vi "General.vi"() -> ()   [LabVIEW 2023]
panel:
  in  "Stop Button":bool
  out "Boolean":bool
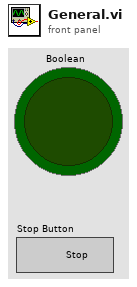
[diagram p1: front panel]
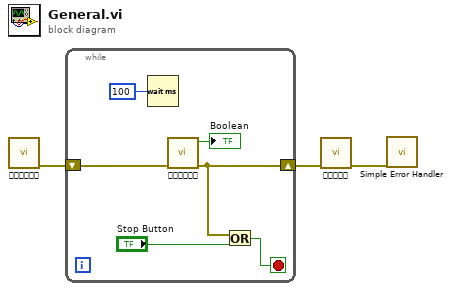
[diagram p0: block diagram]
diagram:
  n1 = call "설정.vi"() -> ("error out"=w3:errorcluster)  [unwired: 11 in]
  n2 = while {
    shift-right: [w6] -> w2
    shift-left: w3 -> [w9]
    stop <- w5 stop-if-true
    n3 = Wait (ms)(milliseconds to wait=u32 100) -> ()  [unwired: 1 out]
    n4 = call "측정.vi"("error in"=w9) -> ("error out"=w6:errorcluster, "Boolean"=→"Boolean":bool)  [unwired: 9 in]
    n5 = Or(x=w6, y="Stop Button") -> (x .or. y?=w5:bool)
  }
  n6 = call "종료.vi"("error in"=w2) -> ("error out"=w1:errorcluster)  [unwired: 10 in]
  n7 = call <vilib>:"Simple Error Handler.vi"("error in (no error)"=w1) -> ()  [unwired: 4 in, 5 out]
